vi "LR-Determine-stable.vi"(7 "Stable level settings":T2, 8 "error in (no error)":errorcluster, 9 "Power in":dbl[](array[numeric]), 11 "Results in":T1) -> (0 "error out":errorcluster, 1 "Power":dbl[](array[numeric]), 3 "Results":T1, 4 "Valid?":bool)   [LabVIEW 2013, in "HardwareCharacterization.lvlib" / "HC-LaserResponse.lvclass"]
doc: "Use this template to build a VI to use as a subVI."
uses:
  HC-LaserResponse.lvclass
  Settings-stable.ctl
  Test-results.ctl
  <vilib>/Analysis/baseanly.llb/Mean (DBL).vi
  <vilib>/Analysis/NI_AALBase.lvlib
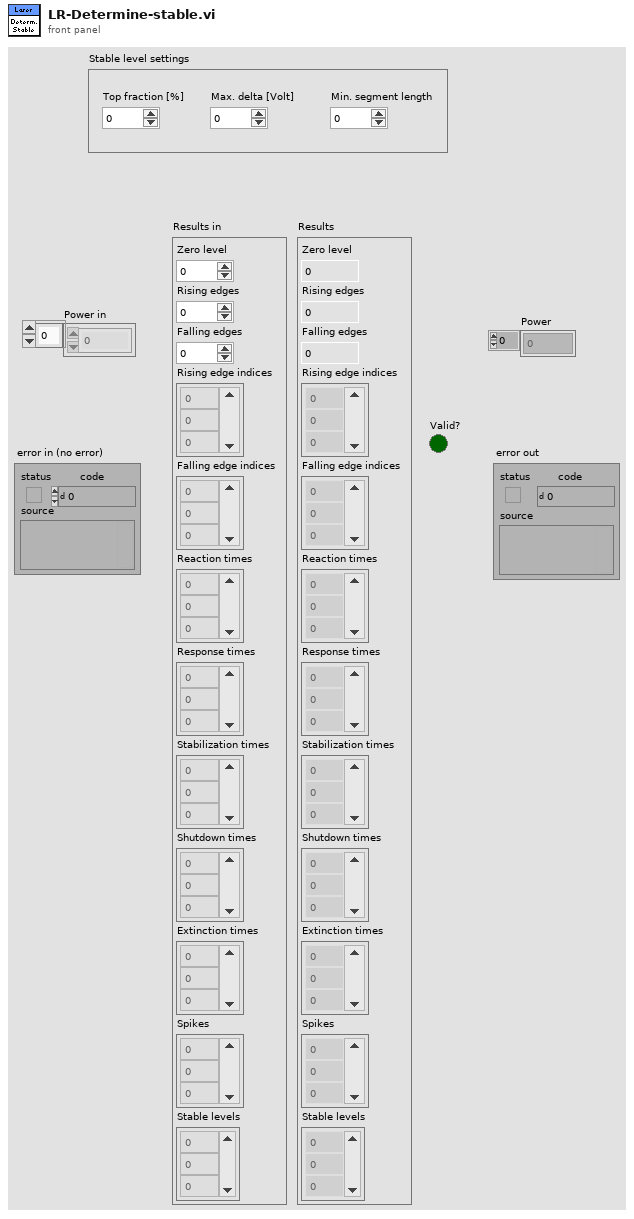
[diagram p1: front panel]
types:
  T1 = typedef "HardwareCharacterization.lvlib/HC-LaserResponse.lvclass/Test-results.ctl" = cluster{"Zero level":dbl, "Rising edges":i32, "Falling edges":i32, "Rising edge indices":dbl[], "Falling edge indices":dbl[], "Reaction times":dbl[], "Response times":dbl[], "Stabilization times":dbl[], "Shutdown times":dbl[], "Extinction times":dbl[], "Spikes":i32[], "Stable levels":dbl[]}
  T2 = typedef "HardwareCharacterization.lvlib/HC-LaserResponse.lvclass/Settings-stable.ctl" = cluster{"Top fraction [%]":i32, "Max. delta [Volt]":dbl, "Min. segment length":i32}
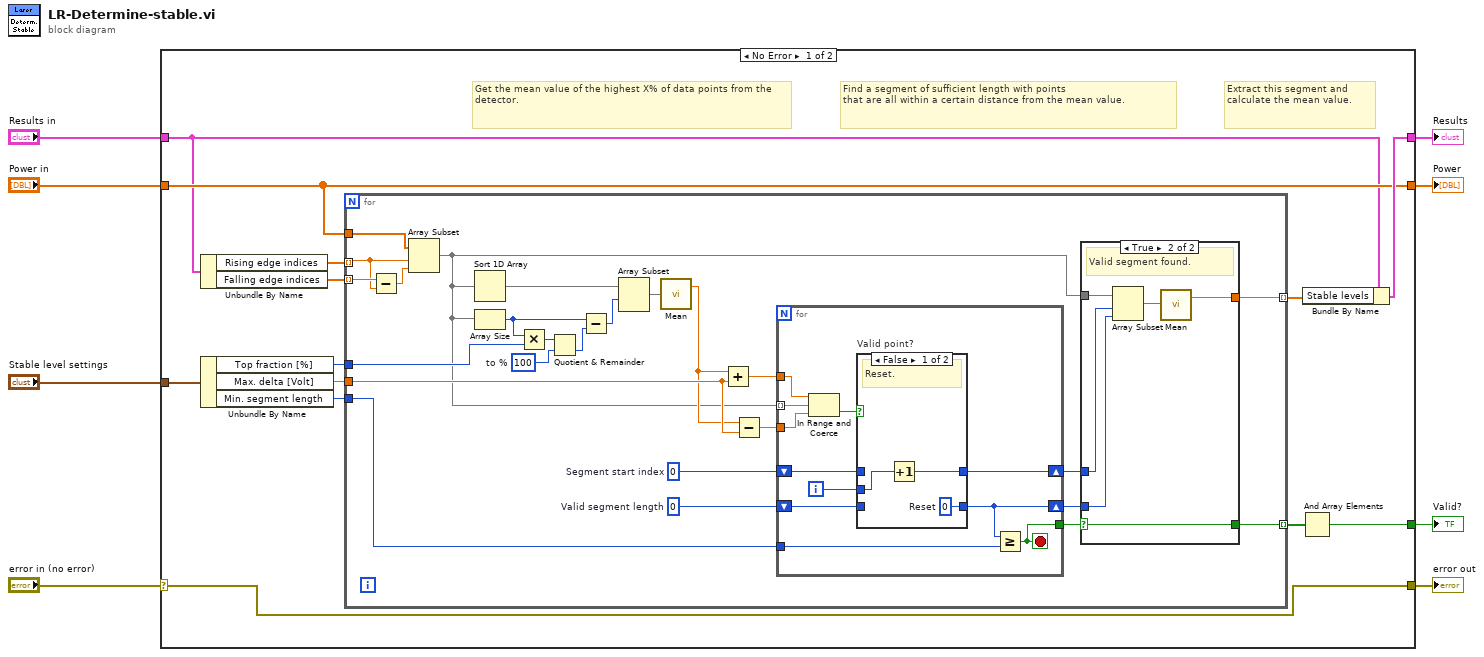
[diagram p0: block diagram]
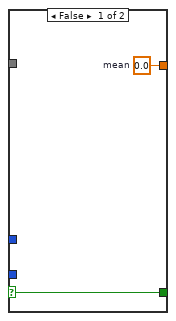
[diagram p2: hidden frame]
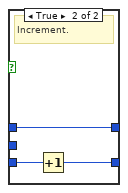
[diagram p3: hidden frame]
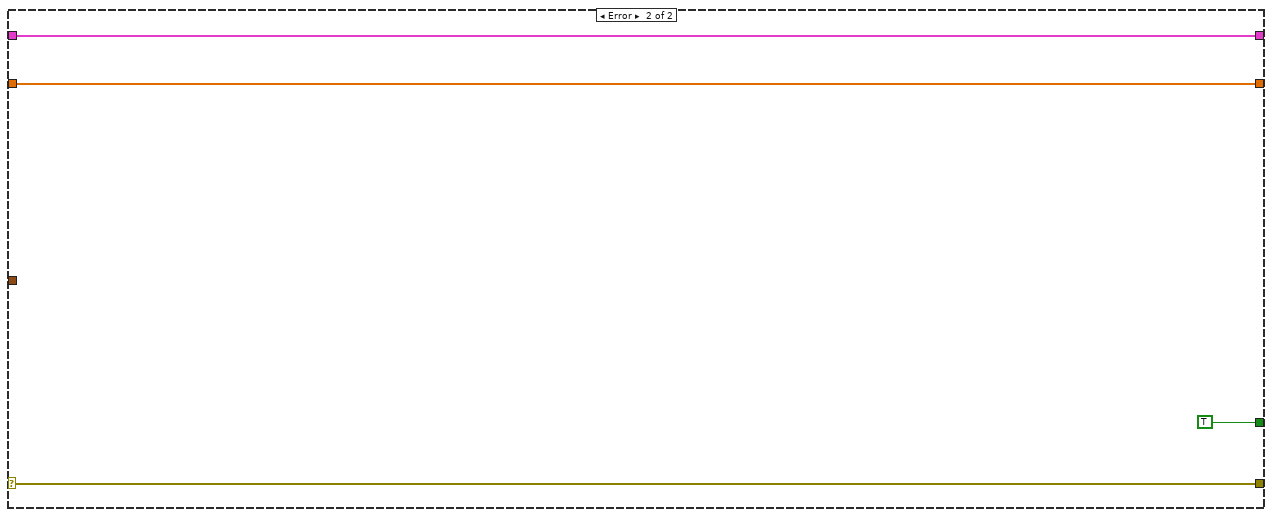
[diagram p4: hidden frame]
diagram:
  n1 = case shown="No Error" "error in (no error)" {
    selector: "error in (no error)" -> [w18 w75]
    tunnel: [w18 w75] -> w7
    tunnel: "Stable level settings" -> [w21 _]
    tunnel: [w9 TRUE] -> w5
    tunnel: "Power in" -> [w13 w73]
    tunnel: [w13 w73] -> w3
    tunnel: "Results in" -> [w12 w72]
    tunnel: [w15 w72] -> w1
    frame No Error {
      # "Extract this segment and \ncalculate the mean value."
      # "Find a segment of sufficient length with points \nthat are all within a certain distance from the mean value."
      # "Get the mean value of the highest X% of data points from the detector."
      n2 = Unbundle By Name(w12) -> ("Rising edge indices"=w11:dbl[], "Falling edge indices"=w10:dbl[])
      n3 = Unbundle By Name(w21) -> ("Top fraction [%]"=w16:i32, "Max. delta [Volt]"=w19:dbl, "Min. segment length"=w20:i32)
      n4 = for {
        tunnel: w20 -> [w43]
        tunnel: w19 -> [w40]
        tunnel: [w34] -> w17 mode=indexing
        tunnel: w16 -> [w29]
        tunnel: [w27] -> w14 mode=indexing
        tunnel: w13 -> [w23]
        tunnel: w11 -> [w24] mode=indexing
        tunnel: w10 -> [w26] mode=indexing
        w38 = 0  # Segment start index
        w44 = 0  # Valid segment length
        w28 = 100  # to %
        n5 = Subtract(x=w26, y=w24) -> (x-y=w25:dbl)
        n6 = Array Subset(array=w23, index=w24, length=w25) -> (w22:dbl[])
        n7 = Sort 1D Array(array=w22) -> (sorted array=w46:dbl[])
        n8 = Array Size(array=w22) -> (size(s)=w31:i32)
        n9 = Multiply(x=w31, y=w29) -> (x*y=w45:i32)
        n10 = Quotient & Remainder(x=w45, y=w28) -> (floor(x/y)=w32:i32)  [unwired: 1 out]
        n11 = Subtract(x=w31, y=w32) -> (x-y=w30:i32)
        n12 = Array Subset(array=w46, index=w30) -> (w39:dbl[])  [unwired: 1 in]
        n13 = call-poly <vilib>:"Mean.vi"("X"=w39) -> ("mean"=w33:dbl)  [unwired: 1 out]
        n14 = Add(x=w33, y=w40) -> (x+y=w42:dbl)
        n15 = Subtract(x=w33, y=w40) -> (x-y=w41:dbl)
        n16 = for {
          shift-right: [w56] -> w37
          shift-left: w44 -> [w61]
          tunnel: w43 -> [w57]
          tunnel: w42 -> [w64]
          tunnel: w41 -> [w63]
          tunnel: w22 -> [w65] mode=indexing
          shift-right: [w58] -> w35
          shift-left: w38 -> [w59]
          tunnel: [w55] -> w36
          i -> [w60]
          stop <- w55 stop-if-true
          n17 = In Range and Coerce(upper limit=w64, x=w65, lower limit=w63) -> (In Range?=w62:bool)  [unwired: 1 out]
          n18 = case "Valid point?" shown="False" w62 {
            tunnel: w61 -> [_ w71]
            tunnel: [w68 w70] -> w56
            tunnel: w60 -> [w67 _]
            tunnel: w59 -> [_ w69]
            tunnel: [w66 w69] -> w58
            frame False {
              w68 = 0  # Reset
              # "Reset."
              n19 = Increment(x=w67) -> (x+1=w66:i32)
            }
            frame True {
              # "Increment."
              n20 = Increment(x=w71) -> (x+1=w70:i32)
            }
          }
          n21 = Greater Or Equal?(x=w56, y=w57) -> (x >= y?=w55:bool)
        }
        n22 = case shown="True" w36 {
          selector: w36 -> [w47 w49]
          tunnel: w37 -> [_ w54]
          tunnel: w22 -> [_ w53]
          tunnel: w35 -> [_ w52]
          tunnel: [w48 w50] -> w27
          tunnel: [w47 w49] -> w34
          frame False {
            w48 = 0.0  # mean
          }
          frame True {
            # "Valid segment found."
            n23 = Array Subset(array=w53, index=w52, length=w54) -> (w51:dbl[])
            n24 = call-poly <vilib>:"Mean.vi"("X"=w51) -> ("mean"=w50:dbl)  [unwired: 1 out]
          }
        }
      }
      n25 = And Array Elements(Boolean array=w17) -> (logical AND=w9:bool)
      n26 = Bundle By Name(cluster=w12, "Stable levels"=w14) -> (w15:T1)
    }
    frame Error {
    }
  }
  "error out" <- w7
  "Valid?" <- w5
  "Power" <- w3
  "Results" <- w1
